vi "matlabtest.vi"() -> ()   [LabVIEW 2013]
panel:
  out "1-D Array of Real":dbl[](array[numeric])
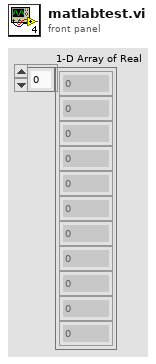
[diagram p1: front panel]
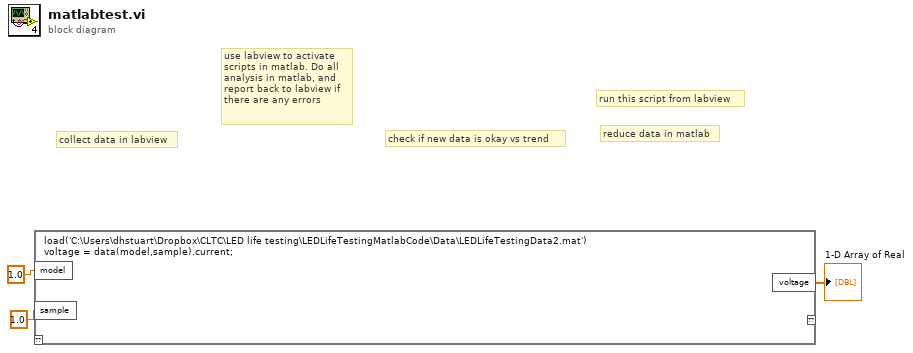
[diagram p0: block diagram]
diagram:
  # "use labview to activate\nscripts in matlab. Do all\nanalysis in matlab, and \nreport back to labview if\nthere are any errors"
  # "check if new data is okay vs trend"
  # "run this script from labview"
  # "reduce data in matlab"
  # "collect data in labview"
  n1 = script code="load('C:\\Users\\dhstuart\\Dropbox\\CLTC\\LED life testing\\LEDLifeTestingMatlabCode\\Data\\LEDLifeTestingData2.mat')\nvoltage = data(model,sample).current;"("model"=1.0 ("Real"), "sample"=1.0 ("Real")) -> ("voltage"=→"1-D Array of Real":dbl[])  [unwired: 1 in, 1 out]
